vi "Intensity Graph and Chart Data Types.vi"() -> ()   [LabVIEW 2018]
doc: "This VI shows the difference between the intensity chart and the intensity graph. It generates a 2D array of random values passes it to the Intensity Graph and Intensity Chart. The Intensity Graph maps 2D data to colors according to its Z scale. The graph draws the most recent data and has no memory of previous data. The Intensity Chart maps data in the same way, but keeps a history. With the scroll bar it is possible to look back through the history."
panel:
  in  "Stop":bool
  out "Intensity Chart":dbl[][](graph)
  out "Intensity Graph":dbl[][](graph)
  # "Overview: Illustrates the data types that can be wired to Intensity Graphs and Intensity Charts.\nInstructions:\n1. Run the VI. Observe the data being displayed in the intensity graph and intensity chart.\n2. Click Stop to stop the VI.\n3. Scroll through the history of the Intensity Chart with its scrollbar."
  # "The Intensity Graph displays an individual set of data with no history. The Intensity Chart keeps a history of the data it has displayed. Right-click the Intensity Chart and select Chart History Length to modify the amount of history data the chart retains."
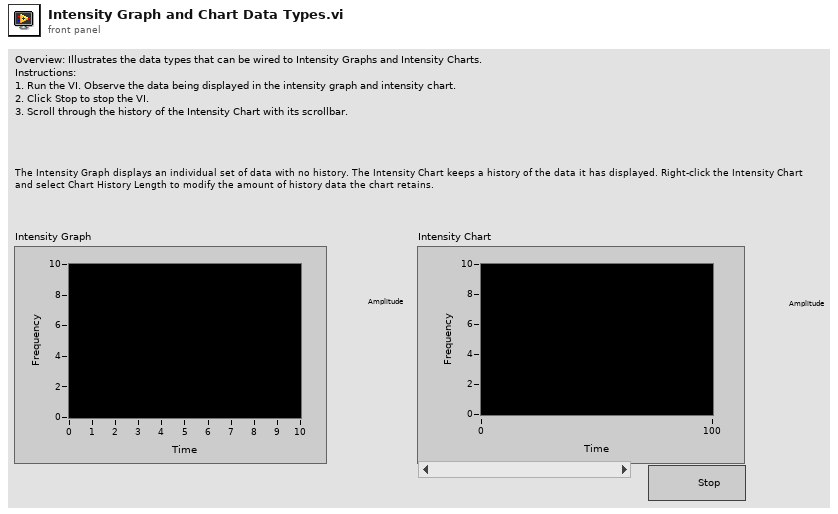
[diagram p1: front panel]
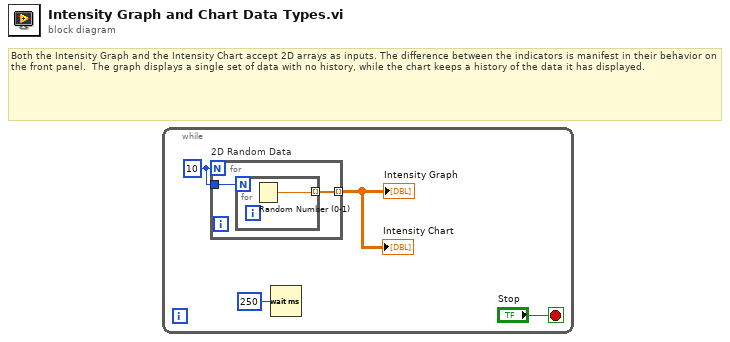
[diagram p0: block diagram]
diagram:
  # "Both the Intensity Graph and the Intensity Chart accept 2D arrays as inputs. The difference between the indicators is manifest in their behavior on the front panel.  The graph displays a single set of data with no history, while the chart keeps a history of the data it has displayed."
  n1 = while {
    stop <- "Stop" stop-if-true
    w2 = 10
    n2 = for "2D Random Data" {
      N: w2 -> [_]
      tunnel: w2 -> [w6]
      tunnel: [w5] -> w1 mode=indexing
      n3 = for {
        N: w6 -> [_]
        tunnel: [w7] -> w5 mode=indexing
        n4 = Random Number (0-1)() -> (number: 0 to 1=w7:dbl)
      }
    }
    "Intensity Graph" <- w1
    "Intensity Chart" <- w1
    n5 = Wait (ms)(milliseconds to wait=u32 250) -> ()  [unwired: 1 out]
  }
